vi "get_download_location.vi"(8 "error in (no error)":errorcluster) -> (0 "error out":errorcluster, 3 "download_location":path)   [LabVIEW 2015, in "lv-post-installer.lvlib"]
uses:
  lv-post-installer.lvlib
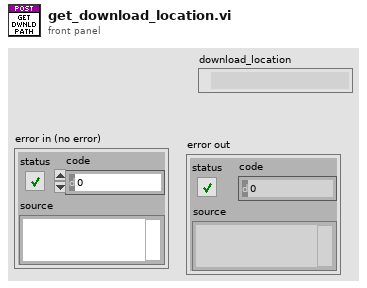
[diagram p1: front panel]
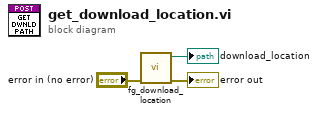
[diagram p0: block diagram]
diagram:
  n1 = call "fg_download_location.vi"("error in (no error)"="error in (no error)") -> ("error out"=→"error out":errorcluster, "path out"=→"download_location":path)  [unwired: 9 in]
